vi "set state.vi"(8 "error in (no error)":errorcluster, 11 "new_state":u32(ring) items=["UNINITIALIZED", "RUNNING", "PAUSED", "EXITING"]) -> (0 "error out":errorcluster, 3 "function return":i32)   [LabVIEW 2014, in "libroboticscape.lvlib"]
doc: "int set_state(state_t new_state);"
uses:
  libroboticscape.lvlib
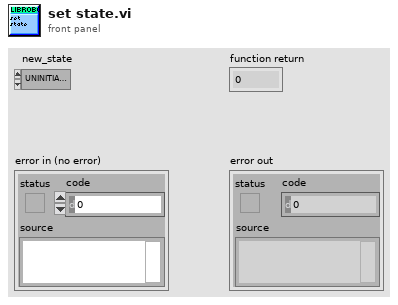
[diagram p1: front panel]
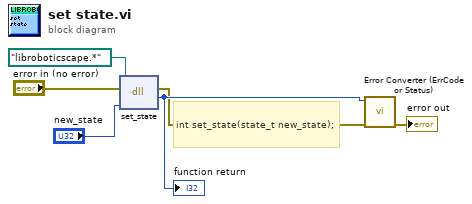
[diagram p0: block diagram]
diagram:
  # "int set_state(state_t new_state);"
  n1 = dll-call lib="C:/Users/ktalke/Documents/Robotics-Cape-Master-Jessie/Libroboticscape-Master-Jessie/libroboticscape.so" fn="set_state"(path in=path "libroboticscape.*", error in="error in (no error)", "new_state"="new_state") -> (error out=w3:errorcluster, "return type"=w6:i32)  [unwired: 2 in, 1 out]
  "function return" <- w6
  n2 = call "Error Converter (ErrCode or Status).vi"("error in (no error)"=w3, "error code"=w6) -> ("error out"=→"error out":errorcluster)  [unwired: 9 in]
